vi "Verify VI.vi"(5 "Options":T1, 7 "Test VI (caller)":string, 8 "error in":errorcluster, 10 "Anything":variant) -> (0 "error out":errorcluster, 1 "Failure Message":string, 2 "Passed?":bool)   [LabVIEW 2020]
doc: "Performs an approval test.\n\nThe first call, the test passes and the test data is written to the approved file.\n\nOn subsequent runs the test data is compared to the contents of the approved file.\nIf it is a match, the test passes.\nIf it is not a match, the test fails and the test data is written to the actual file.\n\nAt the point the user can diff the approved and actual files and determine if they approve of the changes or not. If they approve, they replace the old approved file with the actual file. \n\nNOTE: You should keep the approved files in Source Code Control. You should ignore *.actual in your .gitignore file - there is no need to store those."
uses:
  Approval Tests.lvlib
  Reporter/Reporter.lvclass
  Printer/Printer.lvclass
  Options.ctl
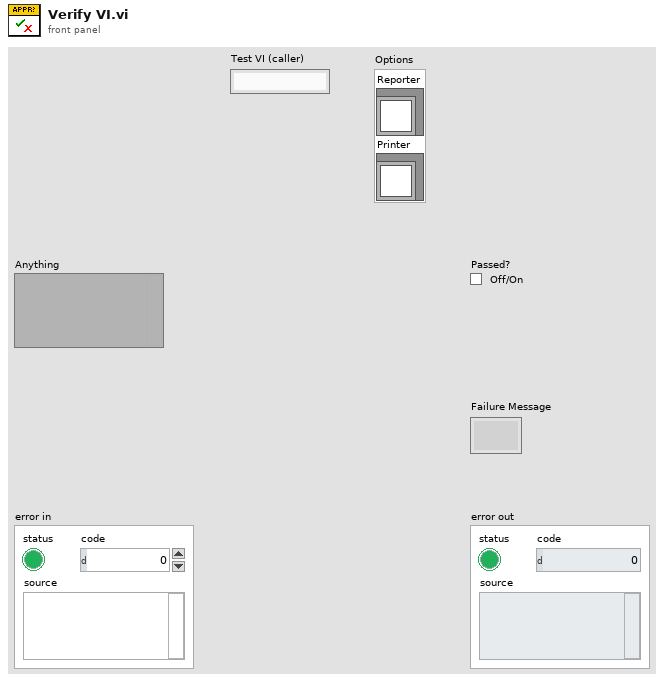
[diagram p1: front panel]
types:
  T1 = typedef "Approval Tests.lvlib/Options.ctl" = cluster{"Reporter":refnum<class "Reporter.lvclass">, "Printer":refnum<class "Printer.lvclass">}
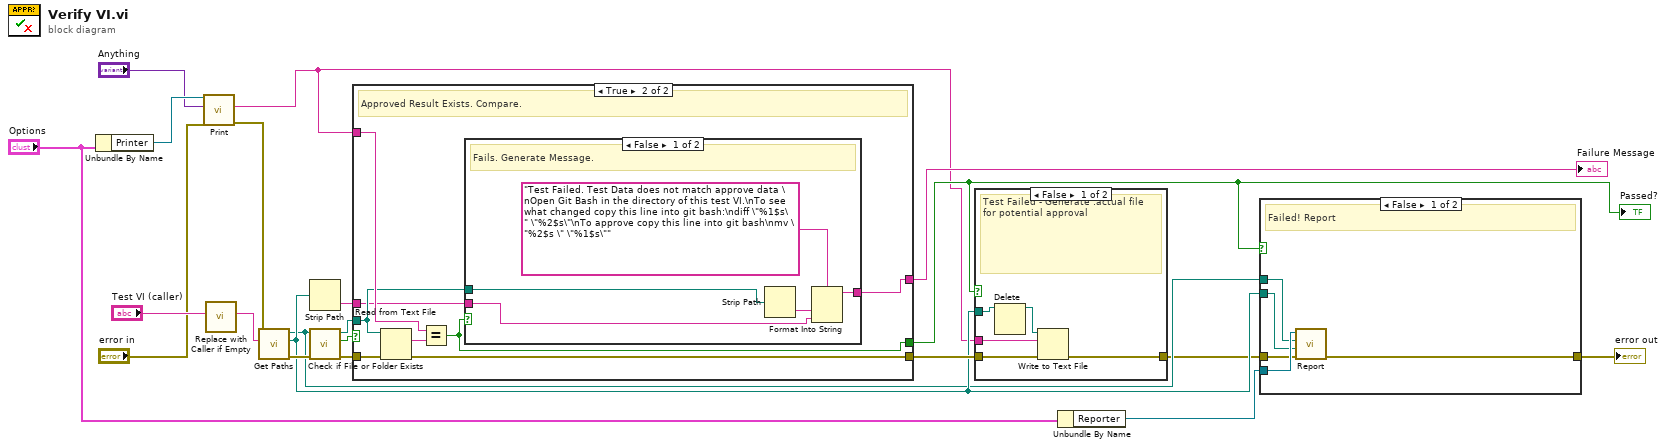
[diagram p0: block diagram]
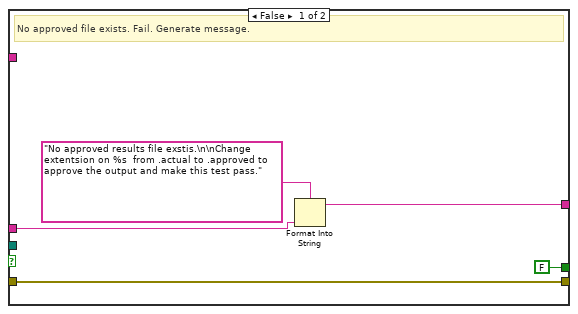
[diagram p4: hidden frame]
diagram:
  n1 = Unbundle By Name("Options") -> ("Printer"=w5:refnum<class "Printer.lvclass">)
  n2 = call-dynamic "Print.vi"("error in (no error)"="error in", "Anything In"="Anything", "Printer in"=w5) -> ("error out"=w1:errorcluster, "Printed String"=w3:string)  [unwired: 6 in, 1 out]
  n3 = call "Replace with Caller if Empty.vi"("Test VI (caller) in"="Test VI (caller)") -> ("Test VI (caller) out"=w10:string)  [unwired: 10 in]
  n4 = call "Get Paths.vi"("error in"=w1, "VI name"=w10) -> ("error out"=w21:errorcluster, "recived path"=w13:path, "approved path"=w12:path)  [unwired: 7 in]
  n5 = Strip Path(path=w13) -> (name=w15:string)  [unwired: 1 out]
  n6 = call <vilib>:"Check if File or Folder Exists.vi"("error in (no error)"=w21, "path"=w12) -> ("error out"=w20:errorcluster, "file or folder exists?"=w17:bool, "dup path"=w18:path)  [unwired: 7 in]
  n7 = case shown="True" w17 {
    tunnel: w3 -> [_ w30]
    tunnel: [w26 w33] -> w19
    tunnel: w20 -> [w26 w34]
    tunnel: w18 -> [_ w28]
    tunnel: [FALSE ("Passed?") w31] -> w14
    tunnel: [w22 w29] -> w16
    tunnel: w15 -> [w24 w27]
    frame False {
      # "No approved file exists. Fail. Generate message."
      n8 = Format Into String(format string="No approved results file exstis.\n\nChange extentsion on %s  from .actual to .approved to approve the output and make this test pass.", w24) -> (resulting string=w22:string)  [unwired: 2 in, 1 out]
    }
    frame True {
      # "Approved Result Exists. Compare."
      n9 = Read from Text File(file (use dialog)=w28, error in=w34) -> (text=w32:string, error out=w33:errorcluster)  [unwired: 2 in, 2 out]
      n10 = Equal?(x=w30, y=w32) -> (x = y?=w31:bool)
      n11 = case shown="False" w31 {
        tunnel: [w39 _] -> w29
        tunnel: w28 -> [w36 _]
        tunnel: w27 -> [w35 _]
        frame False {
          # "Fails. Generate Message."
          n12 = Strip Path(path=w36) -> (name=w37:string)  [unwired: 1 out]
          n13 = Format Into String(format string="Test Failed. Test Data does not match approve data \nOpen Git Bash in the directory of this test VI.\nTo see what changed copy this line into git bash:\ndiff \"%1$s\" \"%2$s\"\nTo approve copy this line into git bash\nmv \"%2$s \" \"%1$s\"", w37, w35) -> (resulting string=w39:string)  [unwired: 2 in, 1 out]
        }
        frame True {
          # "Passes. No Message Needed.."
        }
      }
    }
  }
  "Passed?" <- w14
  "Failure Message" <- w16
  n14 = case shown="False" w14 {
    tunnel: w19 -> [w43 w45]
    tunnel: [w44 w45] -> w9
    tunnel: w13 -> [w42 _]
    tunnel: w3 -> [w40 _]
    frame False {
      # "Test Failed - Generate .actual file for potential approval"
      n15 = Delete(path (use dialog)=w42) -> (deleted path=w41:path)  [unwired: 4 in, 2 out]
      n16 = Write to Text File(file (use dialog)=w41, text=w40, error in=w43) -> (error out=w44:errorcluster)  [unwired: 1 in, 2 out]
    }
    frame True {
      # "Passed - no need for .actual file"
    }
  }
  n17 = Unbundle By Name("Options") -> ("Reporter"=w7:refnum<class "Reporter.lvclass">)
  n18 = case shown="False" w14 {
    tunnel: w13 -> [w48 _]
    tunnel: w12 -> [w49 _]
    tunnel: w7 -> [w50 _]
    tunnel: w9 -> [w47 w51]
    tunnel: [w46 w51] -> w8
    frame False {
      # "Failed! Report"
      n19 = call-dynamic "Report.vi"("error in (no error)"=w47, "Received"=w48, "Approved"=w49, "Reporter in"=w50) -> ("error out"=w46:errorcluster)  [unwired: 6 in, 1 out]
    }
    frame True {
      # "Passed - Nothing to Report"
    }
  }
  "error out" <- w8
